vi "Load Flow Calibration.vi"() -> (0 "CalDate":string, 1 "ATSNumber":string, 2 "GPM Output":dbl[](array[numeric]), 3 "Hz Output":dbl[](array[numeric]))   [LabVIEW 2018]
panel:
  out "Array":string[](array[string])
  out "text":string
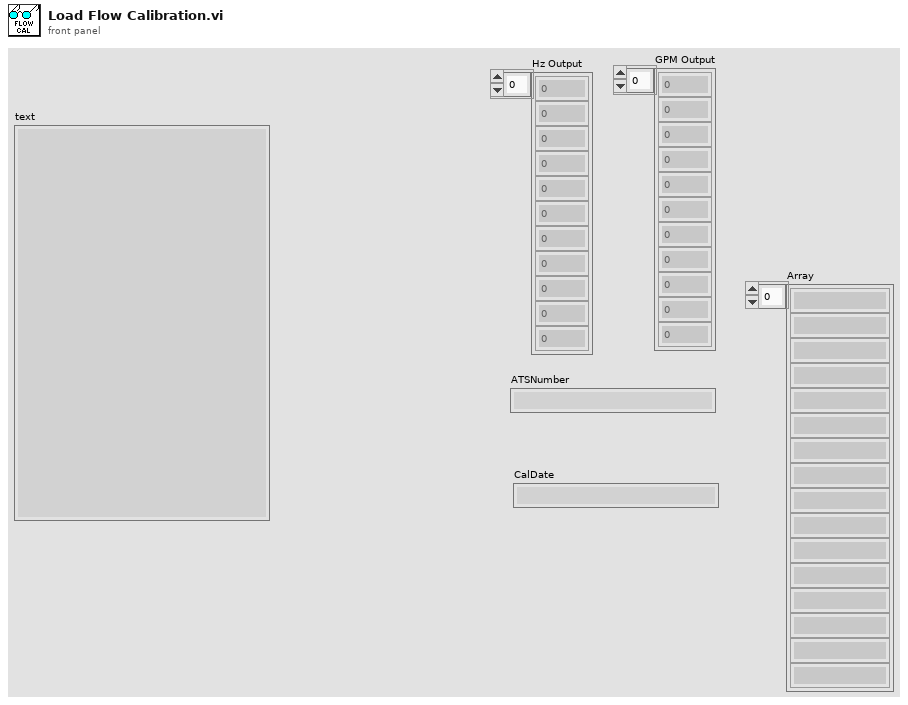
[diagram p1: front panel]
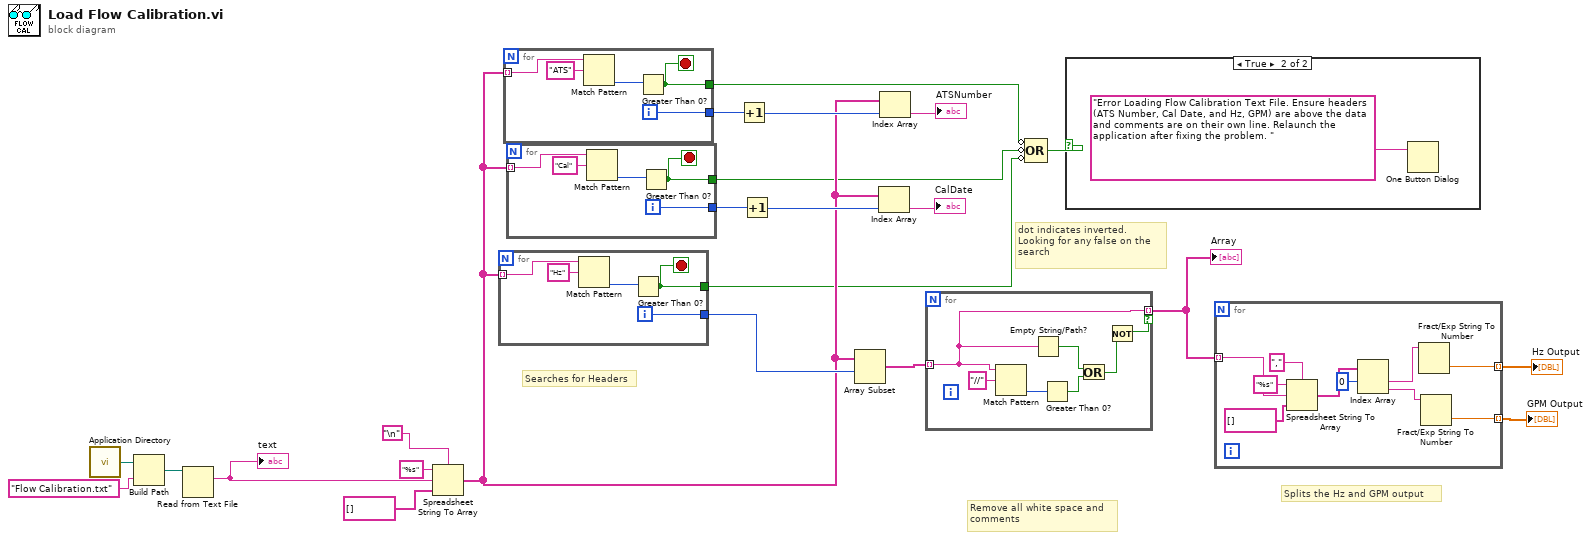
[diagram p0: block diagram]
diagram:
  # "dot indicates inverted. \nLooking for any false on the\nsearch"
  # "Searches for Headers"
  # "Splits the Hz and GPM output"
  # "Remove all white space and\ncomments"
  n1 = call <vilib>:"Application Directory.vi"() -> ("Application Directory"=w21:path)
  n2 = Build Path(base path=w21, name or relative path="Flow Calibration.txt") -> (appended path=w22:path)
  n3 = Read from Text File(file (use dialog)=w22) -> (text=w19:string)  [unwired: 3 in, 3 out]
  "text" <- w19
  n4 = Spreadsheet String To Array(delimiter (Tab)="\n", format string="%s", spreadsheet string=w19, array type (2D Dbl)=string[] []) -> (array=w7:string[])
  n5 = for {
    tunnel: w7 -> [w26] mode=indexing
    tunnel: [w25] -> w2
    tunnel: [w24] -> w15
    i -> [w24]
    stop <- w25 stop-if-true
    n6 = Match Pattern(string=w26, regular expression="Hz") -> (offset past match=w27:i32)  [unwired: 1 in, 3 out]
    n7 = Greater Than 0?(x=w27) -> (x > 0?=w25:bool)
  }
  n8 = for {
    tunnel: w7 -> [w31] mode=indexing
    tunnel: [w30] -> w4
    tunnel: [w29] -> w16
    i -> [w29]
    stop <- w30 stop-if-true
    n9 = Match Pattern(string=w31, regular expression="ATS") -> (offset past match=w32:i32)  [unwired: 1 in, 3 out]
    n10 = Greater Than 0?(x=w32) -> (x > 0?=w30:bool)
  }
  n11 = for {
    tunnel: w7 -> [w36] mode=indexing
    tunnel: [w35] -> w3
    tunnel: [w34] -> w8
    i -> [w34]
    stop <- w35 stop-if-true
    n12 = Match Pattern(string=w36, regular expression="Cal") -> (offset past match=w37:i32)  [unwired: 1 in, 3 out]
    n13 = Greater Than 0?(x=w37) -> (x > 0?=w35:bool)
  }
  n14 = Increment(x=w16) -> (x+1=w13:i32)
  n15 = Increment(x=w8) -> (x+1=w9:i32)
  n16 = Array Subset(array=w7, index=w15) -> (w14:string[])  [unwired: 1 in]
  n17 = Index Array(array=w7, index=w9) -> (element=→"CalDate":string)
  n18 = Index Array(array=w7, index=w13) -> (element=→"ATSNumber":string)
  n19 = for {
    tunnel: w14 -> [w41] mode=indexing
    tunnel: [w41] -> w11 mode=indexing if=w39
    n20 = Match Pattern(string=w41, regular expression="//") -> (offset past match=w44:i32)  [unwired: 1 in, 3 out]
    n21 = Empty String/Path?(string/path=w41) -> (empty?=w42:bool)
    n22 = Greater Than 0?(x=w44) -> (x > 0?=w43:bool)
    n23 = Or(x=w42, y=w43) -> (x .or. y?=w40:bool)
    n24 = Not(x=w40) -> (.not. x?=w39:bool)
  }
  "Array" <- w11
  n25 = Compound Arithmetic op=OR(invert w4, invert w3, invert w2) -> (w1:bool)
  n26 = case shown="True" w1 {
    frame False {
    }
    frame True {
      n27 = One Button Dialog(message="Error Loading Flow Calibration Text File. Ensure headers (ATS Number, Cal Date, and Hz, GPM) are above the data and comments are on their own line. Relaunch the application after fixing the problem. ") -> ()  [unwired: 1 in, 1 out]
    }
  }
  n28 = for {
    tunnel: w11 -> [w56] mode=indexing
    tunnel: [w49] -> w6 mode=indexing
    tunnel: [w47] -> w5 mode=indexing
    n29 = Spreadsheet String To Array(delimiter (Tab)=",", format string="%s", spreadsheet string=w56, array type (2D Dbl)=string[] []) -> (array=w54:string[])
    n30 = Index Array(array=w54, index #1=0 ("index (row)")) -> (element #1=w50:string, element #2=w48:string)  [unwired: 1 in]
    n31 = Fract/Exp String To Number(string=w50) -> (number=w49:dbl)  [unwired: 3 in, 1 out]
    n32 = Fract/Exp String To Number(string=w48) -> (number=w47:dbl)  [unwired: 3 in, 1 out]
  }
  "Hz Output" <- w6
  "GPM Output" <- w5
